vi "Check.vi"() -> ()   [LabVIEW 2019]
uses:
  Y.xctl
  Heating/ctl/Y_source.ctl
  11e5243e-5a90-4a18-a517-0b9e63bafbe7.vi
  95228b63-dbad-4f81-a48d-2b4403cca3b5.vi
  Heating/Heating.lvlib
panel:
  in  "SP_Source":T1
  in  "Y":T2(xcontrol)
  in  "scale max":dbl
  out "Numeric 3":dbl
  out "Numeric 2":dbl
  out "Numeric":dbl
  in  "SP":dbl
  in  "SP_Set":dbl
  in  "connect":bool
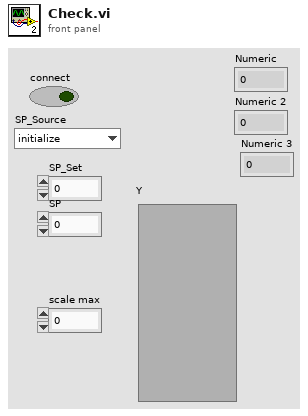
[diagram p1: front panel]
types:
  T1 = typedef "Heating.lvlib/Y_source.ctl" = enum8{"initialize", "local disabled", "local hand", "hand", "auto", "dist"}
  T2 = cluster{"Numeric":dbl, "Numeric":dbl, "Numeric":dbl}
  T3 = cluster{"connect":bool, "SP_Source":T1, "SP_Set":dbl, "SP":dbl}
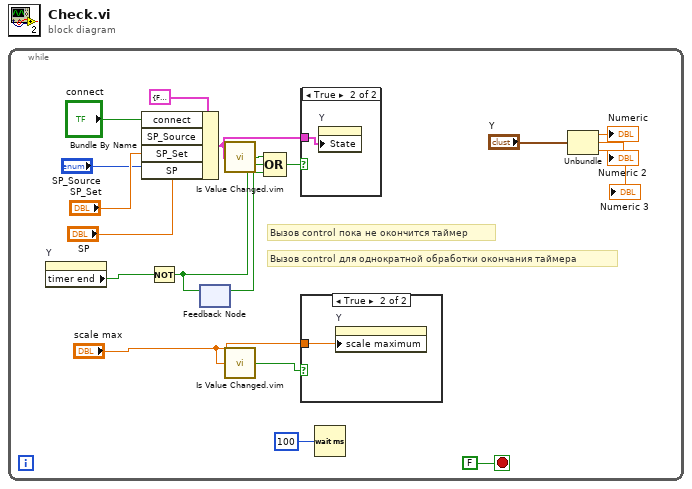
[diagram p0: block diagram]
diagram:
  n1 = while {
    stop <- FALSE stop-if-true
    # "Вызов control пока не окончится таймер"
    # "Вызов control для однократной обработки окончания таймера"
    n2 = property on="Y" class="Y (strict)"() -> ("timer end"=w1:bool)  [unwired: 2 in, 2 out]
    n3 = Bundle By Name(cluster=T3 {"connect"=FALSE, "SP_Source"=enum."initialize", "SP_Set"=0.0, "SP"=0.0} ("source"), "connect"="connect", "SP_Source"="SP_Source", "SP_Set"="SP_Set", "SP"="SP") -> (w7:T3)
    n4 = Not(x=w1) -> (.not. x?=w15:bool)
    n5 = feedback-in #1(w15) -> ()
    n6 = feedback #1() -> (w16:bool)  [unwired: 1 in]
    n7 = call "Is Value Changed.vim"("value"=w7) -> ("changed or first call?"=w13:bool)
    n8 = call "Is Value Changed.vim"("value"="scale max") -> ("changed or first call?"=w5:bool)
    n9 = Compound Arithmetic op=OR(w13, w15, w16) -> (w17:bool)
    n10 = case shown="True" w17 {
      tunnel: w7 -> [_ w21]
      frame False {
      }
      frame True {
        n11 = property on="Y" class="Y (strict)"("State"=w21) -> ()  [unwired: 2 in, 2 out]
      }
    }
    n12 = case shown="True" w5 {
      tunnel: "scale max" -> [_ w20]
      frame False {
      }
      frame True {
        n13 = property on="Y" class="Y (strict)"("scale maximum"=w20) -> ()  [unwired: 2 in, 2 out]
      }
    }
    n14 = Wait (ms)(milliseconds to wait=u32 100) -> ()  [unwired: 1 out]
    n15 = Unbundle("Y") -> ("Numeric"=→"Numeric":dbl, "Numeric"=→"Numeric 2":dbl, "Numeric"=→"Numeric 3":dbl)
  }
